vi "STOP.vi"(8 "error in (no error)":errorcluster, 11 "Stop in":refnum<class "OWIS_TANGO.lvclass">) -> (0 "error out":errorcluster, 3 "Stop out":refnum<class "OWIS_TANGO.lvclass">)   [LabVIEW 2020, in "OWIS_TANGO.lvclass"]
uses:
  OWIS_TANGO.lvclass
  DelayLine.lvclass
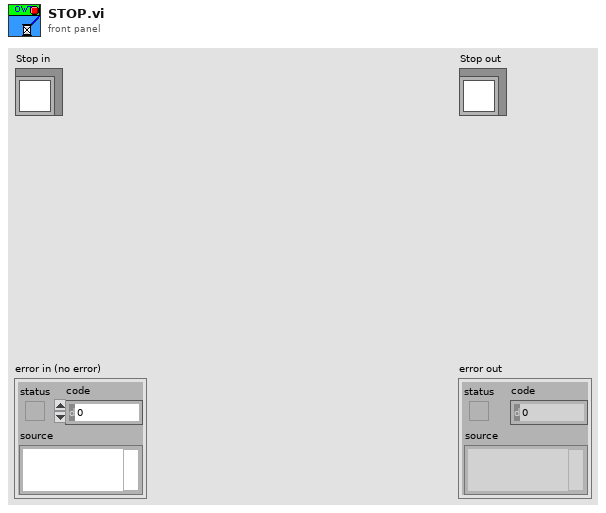
[diagram p1: front panel]
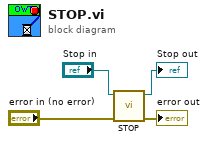
[diagram p0: block diagram]
diagram:
  n1 = call-parent "STOP.vi"("error in (no error)"="error in (no error)", "Stop in"="Stop in") -> ("error out"=→"error out":errorcluster, "Stop out"=→"Stop out":refnum<class "OWIS_TANGO.lvclass">)  [unwired: 8 in]
